vi "Example.vi"() -> ()   [LabVIEW 2022 SP3]
uses:
  usbtmc_scpi_labtool.lvlib
panel:
  in  "Exit on apply (F: Off)":bool
  in  "Apply Settings":bool
  in  "VISA resource name in":refnum<visa-resource-name>="USB0::0xCAFE::0x4000::123456::INSTR"
  in  "Pin":u8 max=7 step=1
  in  "Enable Input Terminal (F: Off)":bool
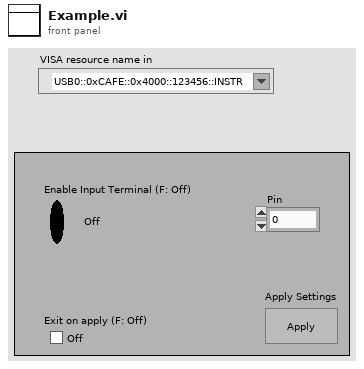
[diagram p1: front panel]
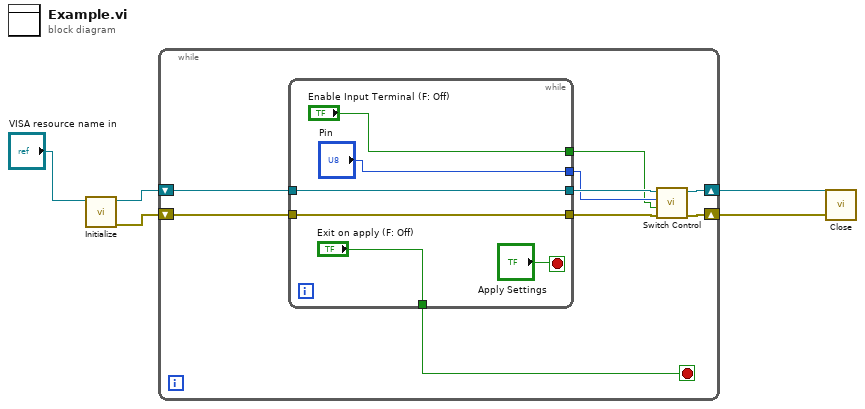
[diagram p0: block diagram]
diagram:
  n1 = call "Initialize.vi"("VISA resource name in"="VISA resource name in") -> ("error out"=w3:errorcluster, "VISA resource name out"=w5:refnum<visa-resource-name>)  [unwired: 9 in]
  n2 = while {
    shift-right: [w14] -> w4
    shift-left: w5 -> [w12]
    shift-right: [w13] -> w2
    shift-left: w3 -> [w11]
    stop <- w6 stop-if-true
    n3 = while {
      tunnel: w12 -> [w18]
      tunnel: w11 -> [w19]
      tunnel: [w19] -> w10
      tunnel: [w18] -> w9
      tunnel: ["Pin"] -> w8
      tunnel: ["Enable Input Terminal (F: Off)"] -> w7
      tunnel: ["Exit on apply (F: Off)"] -> w6
      stop <- "Apply Settings" stop-if-true
    }
    n4 = call "Switch Control.vi"("VISA resource name"=w9, "Pin"=w8, "Enable Input Terminal (F: Off)"=w7, "error in (no error)"=w10) -> ("VISA resource name out"=w14:refnum<visa-resource-name>, "error out"=w13:errorcluster)  [unwired: 5 in]
  }
  n5 = call "Close.vi"("error in (no error)"=w2, "VISA resource name"=w4) -> ()  [unwired: 10 in]
